vi "KE622x -- Set Meas Event Enable Reg State.vi"(0 "VISA Resource In":refnum<visa-resource-name>, 1 "Error Query (T)?":bool=TRUE, 7 "KE622x Meas Event Enable Reg":T1, 11 "error in (no error)":errorcluster) -> (4 "VISA Resource Out (dupl)":refnum<visa-resource-name>, 15 "error out":errorcluster)   [LabVIEW 2019, in "Keithley 622x.lvlib"]
doc: "Sets the bits in the 'Measurement Event Enable' register of the Status Model. Note that only the used (named) bits are settable -- all other bits default to zero."
uses:
  Keithley 622x.lvlib
  Typedefs/KE622x -- Meas Event Enable Reg State.ctl
panel:
  out "Reg Num (dec)":u16 format="%0d"
  out "Reg Num (binary)":u16 format="%016b"
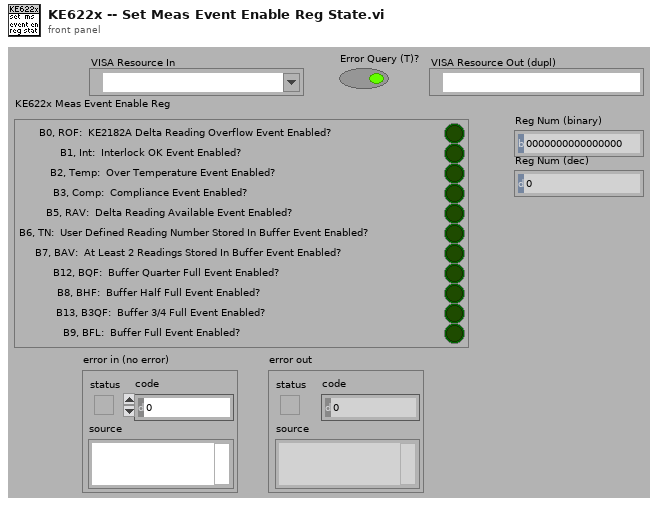
[diagram p1: front panel]
types:
  T1 = typedef "Keithley 622x.lvlib/KE622x -- Meas Event Enable Reg State.ctl" = cluster{"B0, ROF:  KE2182A Delta Reading Overflow Event Enabled?":bool, "B1, Int:  Interlock OK Event Enabled?":bool, "B2, Temp:  Over Temperature Event Enabled?":bool, "B3, Comp:  Compliance Event Enabled?":bool, "B5, RAV:  Delta Reading Available Event Enabled?":bool, "B6, TN:  User Defined Reading Number Stored In Buffer Event Enabled?":bool, "B7, BAV:  At Least 2 Readings Stored In Buffer Event Enabled?":bool, "B12, BQF:  Buffer Quarter Full Event Enabled?":bool, "B8, BHF:  Buffer Half Full Event Enabled?":bool, "B13, B3QF:  Buffer 3/4 Full Event Enabled?":bool, "B9, BFL:  Buffer Full Event Enabled?":bool}
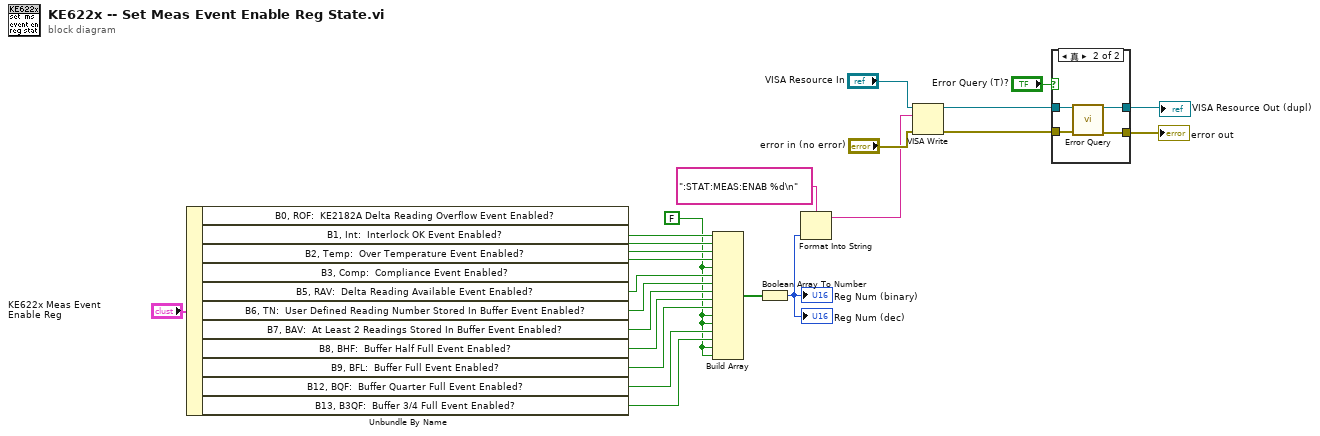
[diagram p0: block diagram]
diagram:
  w1 = FALSE
  n1 = Unbundle By Name("KE622x Meas Event Enable Reg") -> ("B0, ROF:  KE2182A Delta Reading Overflow Event Enabled?"=w12:bool, "B1, Int:  Interlock OK Event Enabled?"=w11:bool, "B2, Temp:  Over Temperature Event Enabled?"=w10:bool, "B3, Comp:  Compliance Event Enabled?"=w9:bool, "B5, RAV:  Delta Reading Available Event Enabled?"=w8:bool, "B6, TN:  User Defined Reading Number Stored In Buffer Event Enabled?"=w7:bool, "B7, BAV:  At Least 2 Readings Stored In Buffer Event Enabled?"=w6:bool, "B8, BHF:  Buffer Half Full Event Enabled?"=w5:bool, "B9, BFL:  Buffer Full Event Enabled?"=w4:bool, "B12, BQF:  Buffer Quarter Full Event Enabled?"=w3:bool, "B13, B3QF:  Buffer 3/4 Full Event Enabled?"=w2:bool)
  n2 = Build Array(w12, w11, w10, w9, w1, w8, w7, w6, w5, w4, w1, w1, w3, w2, w1, w1) -> (w24:bool[])
  n3 = Boolean Array To Number(Boolean array=w24) -> (number=w21:u32)
  "Reg Num (binary)" <- w21
  "Reg Num (dec)" <- w21
  n4 = Format Into String(format string=":STAT:MEAS:ENAB %d\n" ("write buffer"), w21) -> (resulting string=w19:string)  [unwired: 2 in, 1 out]
  n5 = VISA Write(VISA resource name="VISA Resource In", write buffer=w19, error in (no error)="error in (no error)") -> (VISA resource name out=w17:refnum<visa-resource-name>, error out=w18:errorcluster)  [unwired: 1 out]
  n6 = case shown="真" "Error Query (T)?" {
    tunnel: w18 -> [w25 w30]
    tunnel: w17 -> [w26 w29]
    tunnel: [w25 w28] -> w16
    tunnel: [w26 w27] -> w15
    frame False {
    }
    frame True {
      n7 = call "Error Query.vi"("VISA Resource In"=w29, "error in (no error)"=w30) -> ("VISA Resource Out (dupl)"=w27:refnum<visa-resource-name>, "error out"=w28:errorcluster)  [unwired: 10 in, 2 out]
    }
  }
  "VISA Resource Out (dupl)" <- w15
  "error out" <- w16
